vi "checkBeginTimeoutPlay.vi"(8 "error in (no error)":errorcluster, 10 "Game":refnum<class "Game.lvclass">, 11 "TimeoutPlay in":refnum<class "TimeoutPlay.lvclass">) -> (0 "error out":errorcluster, 2 "BeginTimeout?":bool, 3 "TimeoutPlay out":refnum<class "TimeoutPlay.lvclass">)   [LabVIEW 2023, in "TimeoutPlay.lvclass"]
uses:
  TimeoutPlay.lvclass
  Game_class/Game.lvclass
  Referee_class/command_interpreted.ctl
  Game_class/Game.lvclass/Game.ctl
  Referee_class/Referee.lvclass/Referee.ctl
  Game_class/Read Referee.vi
  Game_class/Read EventsRef.vi
  Referee_class/Read command_interpreted.vi
  Referee_class/Referee.lvclass
  Events_class/Events.lvclass
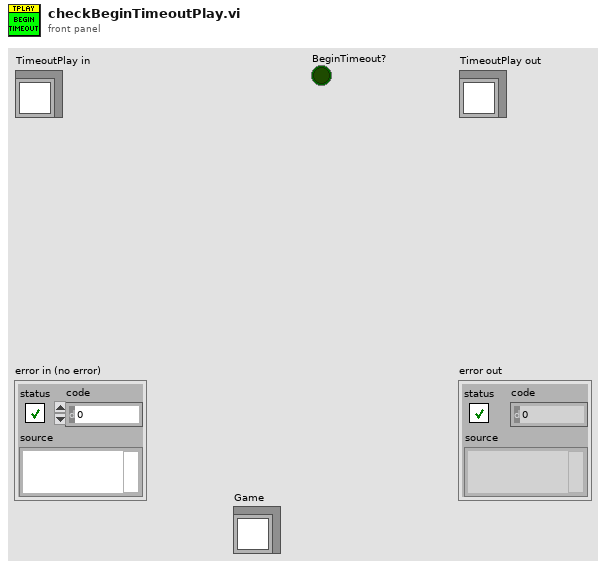
[diagram p1: front panel]
types:
  T1 = typedef "command_interpreted.ctl" = enum16{"Goal Ally", "Goal Enemy", "Ball Placement Enemy", "Ball Placement Ally", "Normal Half Time", "Extra Time  Break", "Extra Half Time", "None", "Post Game", "PKA Normal Start", "Prepare Kickoff Ally", "PKE Normal Start", "Prepare Kickoff Enemy", "Force Start", "Halt", "Timeout", "Prepare Penalty Ally", "Prepare Penalty Enemy", "PPA NormalStart", "PPE Normal Start", "Indirect Free Ally", "Direct Free Enemy", "Direct Free Ally", "Indirect Free Enemy", "Stop"}
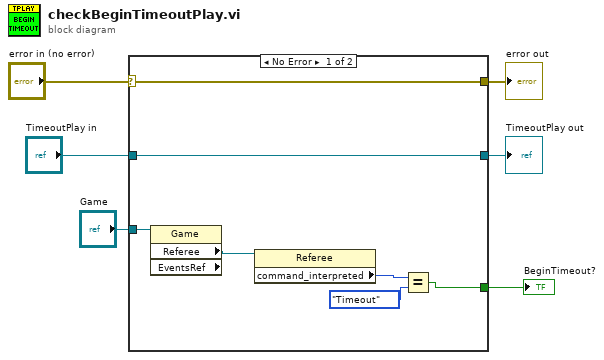
[diagram p0: block diagram]
diagram:
  n1 = case shown="No Error" "error in (no error)" {
    selector: "error in (no error)" -> [w12 w15]
    tunnel: [w12 w15] -> w5
    tunnel: [w13 w14] -> w3
    tunnel: "TimeoutPlay in" -> [w13 w14]
    tunnel: "Game" -> [w8 _]
    tunnel: [w7 _] -> w1
    frame No Error {
      n2 = property class="Game" props=["Referee", "EventsRef"](reference=w8) -> ("Referee"=w11:refnum<class "Referee.lvclass">)  [unwired: 1 in, 3 out]
      n3 = property class="Referee"(reference=w11) -> ("command_interpreted"=w9:T1)  [unwired: 1 in, 2 out]
      n4 = Equal?(x=w9, y=command_interpreted."Timeout" ("command_interpreted")) -> (x = y?=w7:bool)
    }
    frame Error {
    }
  }
  "error out" <- w5
  "TimeoutPlay out" <- w3
  "BeginTimeout?" <- w1
